vi "Convert from String.vi"(8 "error in (no error)":errorcluster, 11 "KA String":string="DB_Query=\"Select\" Connection=\"c:\\Temp\" ") -> (0 "error out":errorcluster, 3 "keyed array":T1)   [LabVIEW 2014, in "Tools_KeyedArray.lvlib"]
uses:
  Tools_KeyedArray.lvlib
  KeyedArray.ctl
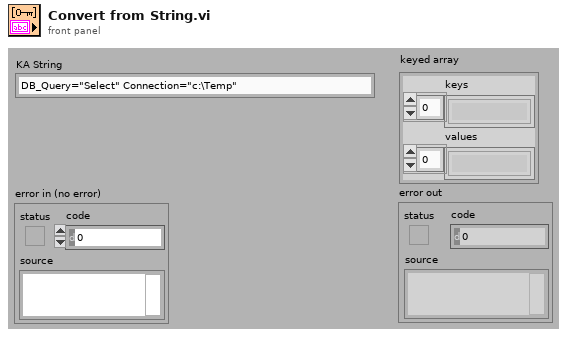
[diagram p1: front panel]
types:
  T1 = typedef "Tools_KeyedArray.lvlib/KeyedArray.ctl" = cluster{"keys":string[], "values":string[]}
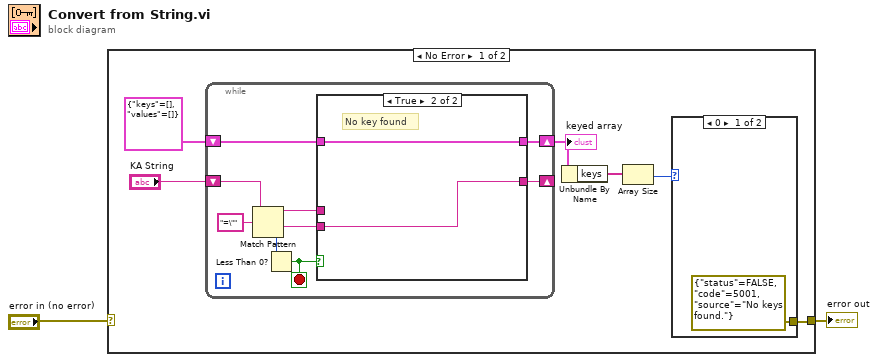
[diagram p0: block diagram]
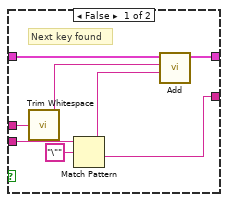
[diagram p3: hidden frame]
diagram:
  n1 = case shown="No Error" "error in (no error)" {
    selector: "error in (no error)" -> [_ w29]
    tunnel: [w3 w29] -> w1
    frame No Error {
      n2 = while {
        shift-right: [w10] -> _
        shift-left: "KA String" -> [w18]
        shift-right: [w12] -> w6
        shift-left: T1 {"keys"=[], "values"=[]} ("keyed array") -> [w13]
        stop <- w15 stop-if-true
        n3 = Match Pattern(string=w18, regular expression="=\"") -> (before substring=w14:string, after substring=w11:string, offset past match=w16:i32)  [unwired: 2 out]
        n4 = Less Than 0?(x=w16) -> (x < 0?=w15:bool)
        n5 = case shown="True" w15 {
          tunnel: w14 -> [w26 _]
          tunnel: w13 -> [w25 w28]
          tunnel: [w24 w28] -> w12
          tunnel: w11 -> [w22 w27]
          tunnel: [w19 w27] -> w10
          frame False {
            # "Next key found"
            n6 = call <vilib>:"Trim Whitespace.vi"("string"=w26) -> ("trimmed string"=w23:string)  [unwired: 1 in]
            n7 = Match Pattern(string=w22, regular expression="\"") -> (before substring=w20:string, after substring=w19:string)  [unwired: 3 out]
            n8 = call "Add.vi"("value"=w20, "key"=w23, "array in"=w25) -> ("array out"=w24:T1)  [unwired: 1 in, 3 out]
          }
          frame True {
            # "No key found"
          }
        }
      }
      "keyed array" <- w6
      n9 = Unbundle By Name(w6) -> ("keys"=w5:string[])
      n10 = Array Size(array=w5) -> (size(s)=w4:i32)
      n11 = case shown="0" w4 {
        tunnel: [errorcluster {"status"=FALSE, "code"=5001, "source"="No keys found."} ("error IO") _] -> w3
        frame 0 {
        }
        frame 1, Default {
        }
      }
    }
    frame Error {
    }
  }
  "error out" <- w1
